vi "Set Neutral Mode.vi"(10 "status":bool, 11 "Enum":enum16{"Coast", "Brake"}(ring)) -> (3 "Motor Control Neutral Mode":u16)   [LabVIEW 2018]
uses:
  <vilib>/Rock Robotics/WPI/ThirdParty/Phoenix-LabVIEW/Motor Controller/Controls/CTRE_Phoenix_MotorControl_NeutralMode.ctl
  <vilib>/Rock Robotics/WPI/ThirdParty/REV Robotics/SPARK MAX/Typedef/Spark MAX Idle Mode.ctl
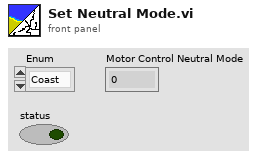
[diagram p1: front panel]
types:
  T1 = typedef "Spark MAX Idle Mode.ctl" = enum16{"Coast", "Brake"}
  T2 = typedef "CTRE_Phoenix_MotorControl_NeutralMode.ctl" = enum8{"EEPROMSetting", "Override to Coast", "Override to Brake"}
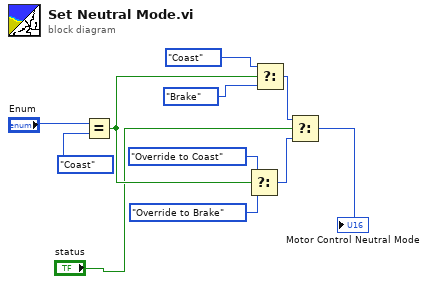
[diagram p0: block diagram]
diagram:
  n1 = Equal?(x="Enum", y=enum16{"Coast", "Brake"}."Coast") -> (x = y?=w4:bool)
  n2 = Select(t=CTRE_Phoenix_MotorControl_NeutralMode."Override to Coast" ("Motor Control Neutral Mode"), s=w4, f=CTRE_Phoenix_MotorControl_NeutralMode."Override to Brake" ("Motor Control Neutral Mode")) -> (s? t:f=w5:T2)
  n3 = Select(t=Spark_MAX_Idle_Mode."Coast" ("Idle Mode"), s=w4, f=Spark_MAX_Idle_Mode."Brake" ("Idle Mode")) -> (s? t:f=w6:T1)
  n4 = Select(t=w6, s="status", f=w5) -> (s? t:f=→"Motor Control Neutral Mode":u16)
